vi "Autonomous Independent.vi"   [LabVIEW 2019]
doc: "This VI is called when autonomous begins, and will automatically be terminated when autonomous ends. You can carry out timed or sensor driven robot movement independently without needing to return to the caller."
uses:
  <vilib>/Rock Robotics/Network Tables/NT Read Number.vi
  Driver Globals.vi
  <vilib>/Rock Robotics/Network Tables/NT Read String.vi
panel:
  # "Be sure to right-click and choose Data Operations>>Make Current Value default if you want to save the array values with the VI"
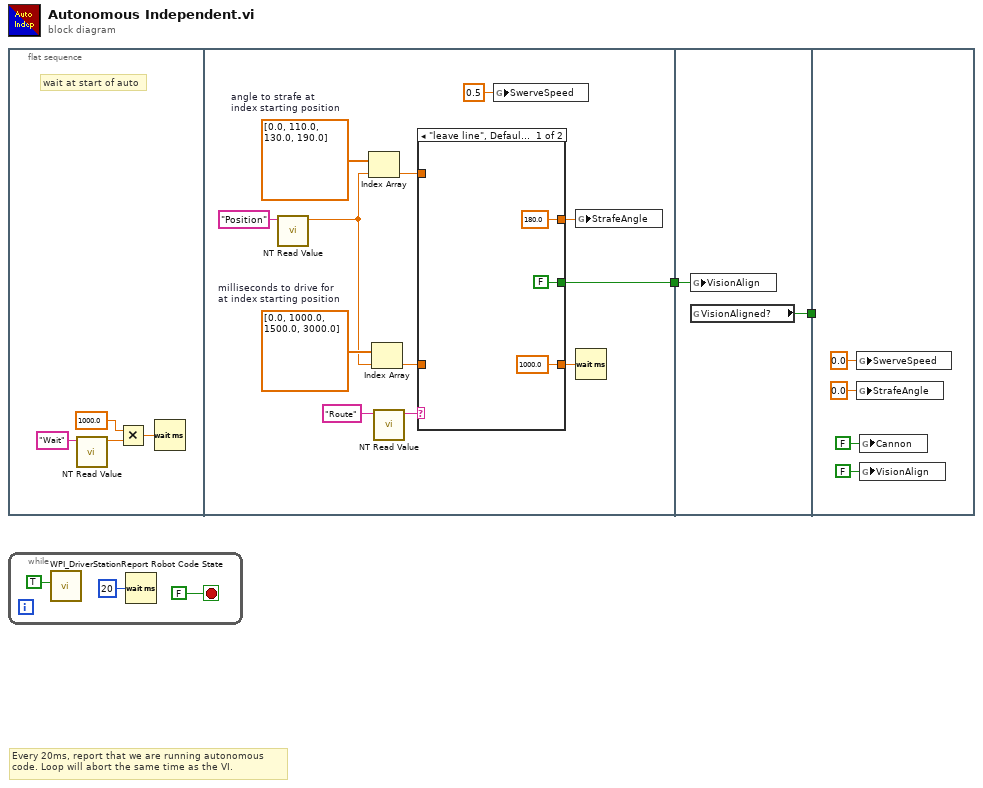
[diagram p0: block diagram]
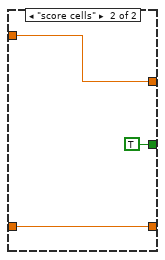
[diagram p2: hidden frame]
diagram:
  # "Every 20ms, report that we are running autonomous\ncode. Loop will abort the same time as the VI."
  n1 = flat-sequence {
    tunnel: [w7] -> w2
    tunnel: w2 -> [w26]
    tunnel: [w25] -> w1
    tunnel: w1 -> [_]
    frame #0 {
      # "wait at start of auto"
      n2 = call-poly <vilib>:"NT Read Value.vi"("Name"="Wait") -> ("Numeric"=w5:dbl)  [unwired: 9 in, 1 out]
      n3 = Multiply(x=1000.0, y=w5) -> (x*y=w4:dbl)
      n4 = Wait (ms)(milliseconds to wait=w4) -> ()  [unwired: 1 out]
    }
    frame #1 {
      w10 = dbl[] [0.0, 1000.0, 1500.0, 3000.0]  # milliseconds to drive for at index starting position
      w16 = dbl[] [0.0, 110.0, 130.0, 190.0]  # angle to strafe at index starting position
      n5 = call-poly <vilib>:"NT Read Value.vi"("Name"="Position") -> ("Numeric"=w9:dbl)  [unwired: 9 in, 1 out]
      n6 = Index Array(array=w16, index=w9) -> (element=w15:dbl)
      n7 = Index Array(array=w10, index=w9) -> (element=w8:dbl)
      n8 = call-poly <vilib>:"NT Read Value.vi"("Name"="Route") -> ("String"=w14:string)  [unwired: 9 in, 1 out]
      n9 = case shown="\"leave line\", Default" w14 {
        tunnel: [180.0 w24] -> w13
        tunnel: w15 -> [_ w24]
        tunnel: [1000.0 w23] -> w11
        tunnel: w8 -> [_ w23]
        tunnel: [FALSE TRUE] -> w7
        frame "leave line", Default {
        }
        frame "score cells" {
        }
      }
      n10 = global write "Driver Globals.vi" "SwerveSpeed"(0.5 ("SwerveSpeed")) -> ()
      n11 = global write "Driver Globals.vi" "StrafeAngle"(w13) -> ()
      n12 = Wait (ms)(milliseconds to wait=w11) -> ()  [unwired: 1 out]
    }
    frame #2 {
      n13 = global write "Driver Globals.vi" "VisionAlign"(w26) -> ()
      n14 = global read "Driver Globals.vi" "VisionAligned?"() -> (w25:bool)
    }
    frame #3 {
      n15 = global write "Driver Globals.vi" "SwerveSpeed"(0.0 ("SwerveSpeed")) -> ()
      n16 = global write "Driver Globals.vi" "StrafeAngle"(0.0 ("StrafeAngle")) -> ()
      n17 = global write "Driver Globals.vi" "Cannon"(FALSE ("Cannon")) -> ()
      n18 = global write "Driver Globals.vi" "VisionAlign"(FALSE ("VisionAlign")) -> ()
    }
  }
  n19 = while {
    stop <- FALSE stop-if-true
    n20 = call <vilib>:"WPI_DriverStationReport Robot Code State.vi"("Autonomous"=TRUE) -> ()  [unwired: 10 in, 1 out]
    n21 = Wait (ms)(milliseconds to wait=u32 20) -> ()  [unwired: 1 out]
  }
